vi "Execute.vi"(8 "error in (no error)":errorcluster, 11 "Action in":refnum<class "Action.lvclass">) -> (0 "error out":errorcluster, 2 "Exit?":bool, 3 "Action out":refnum<class "Action.lvclass">)   [LabVIEW 2018, in "Action.lvclass"]
uses:
  Action.lvclass
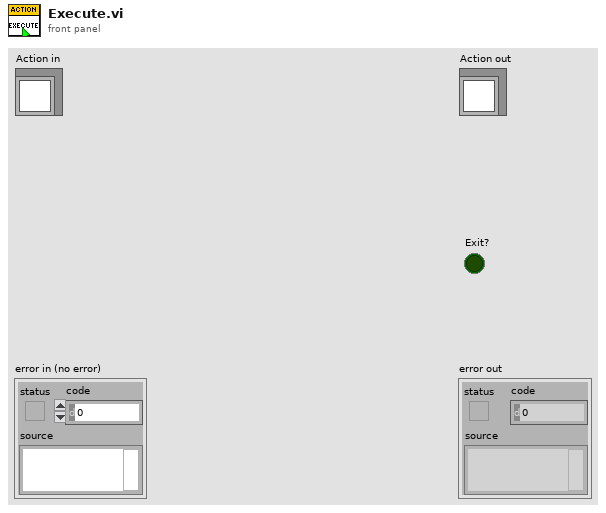
[diagram p1: front panel]
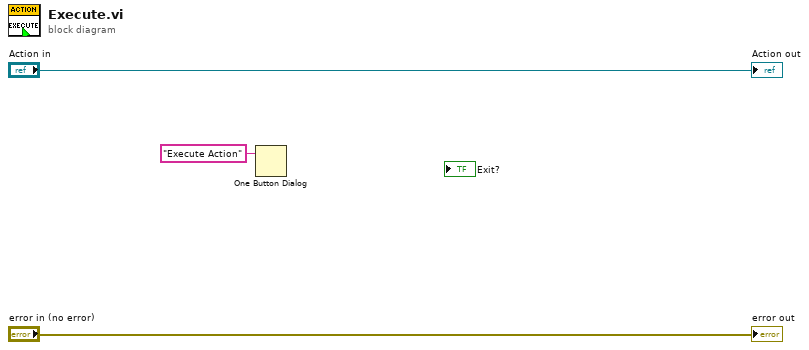
[diagram p0: block diagram]
diagram:
  n1 = One Button Dialog(message="Execute Action") -> ()  [unwired: 1 in, 1 out]
  "error out" <- "error in (no error)"
  "Action out" <- "Action in"
